vi "Configure Trend Scale.vi"(0 "VISA resource name":refnum<visa-resource-name>, 5 "Scale Digit (0 : Normal)":i32(ring) items=["Normal", "Fine"], 7 "Value Display (0 : Mark)":i32(ring) items=["Mark", "Bar graph"], 9 "digit (0: 0-digit)":i32(ring) items=["0-Digit"=0, "3-Digit"=3, "4-Digit"=4], 11 "error in (no error)":errorcluster) -> (4 "VISA resource name out":refnum<visa-resource-name>, 15 "error out":errorcluster)   [LabVIEW 2020, in "Yokogawa GX Series.lvlib"]
doc: "Sets the scale.\n\nCommand: STrdScale\n\nNote: This VI does nothing when the instrument is GM10."
uses:
  <instrlib>/Yokogawa GX Series/Yokogawa GX Series.lvlib
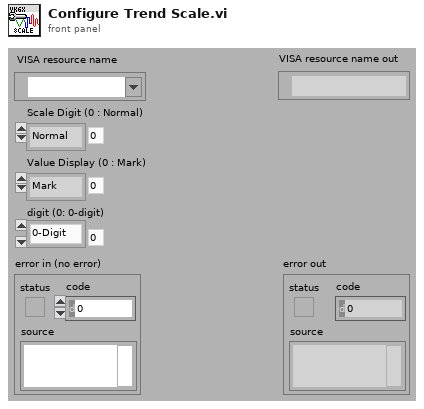
[diagram p1: front panel]
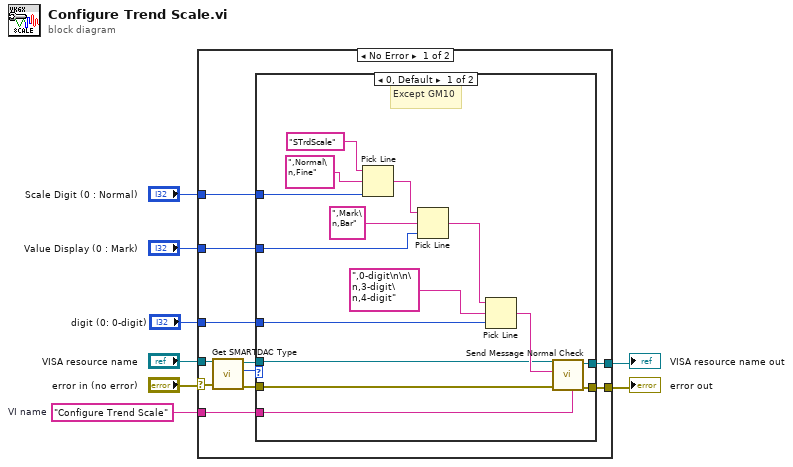
[diagram p0: block diagram]
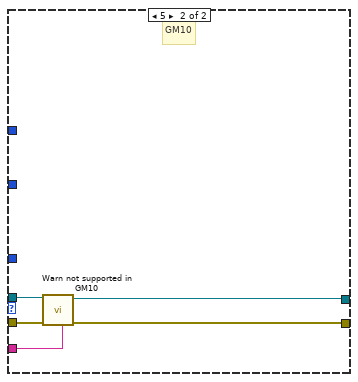
[diagram p2: hidden frame]
diagram:
  w5 = "Configure Trend Scale"  # VI name
  n1 = case shown="No Error" "error in (no error)" {
    selector: "error in (no error)" -> [w12 w40]
    tunnel: "Scale Digit (0 : Normal)" -> [w19 _]
    tunnel: "Value Display (0 : Mark)" -> [w18 _]
    tunnel: "digit (0: 0-digit)" -> [w17 _]
    tunnel: w5 -> [w16 _]
    tunnel: "VISA resource name" -> [w13 w41]
    tunnel: [w15 w41] -> w3
    tunnel: [w14 w40] -> w2
    frame No Error {
      n2 = call <instrlib>:"Get SMARTDAC Type.vi"("error in (no error)"=w12, "VISA resource name"=w13) -> ("error out"=w10:errorcluster, "SMARTDAC+ Type"=w9:u16, "VISA resource name out"=w11:refnum<visa-resource-name>)  [unwired: 7 in]
      n3 = case shown="0, Default" w9 {
        tunnel: w19 -> [w33 _]
        tunnel: w18 -> [w31 _]
        tunnel: w17 -> [w21 _]
        tunnel: w16 -> [w25 w35]
        tunnel: w11 -> [w24 w39]
        tunnel: [w23 w37] -> w15
        tunnel: [w22 w36] -> w14
        tunnel: w10 -> [w20 w38]
        frame 0, Default {
          # "Except GM10"
          n4 = Pick Line(string ("")="STrdScale", multi-line string=",Normal\n,Fine", line index=w33) -> (output string=w30:string)
          n5 = Pick Line(string ("")=w30, multi-line string=",Mark\n,Bar", line index=w31) -> (output string=w28:string)
          n6 = Pick Line(string ("")=w28, multi-line string=",0-digit\n\n\n,3-digit\n,4-digit", line index=w21) -> (output string=w26:string)
          n7 = call <instrlib>:"Send Message Normal Check.vi"("Source (\"\")"=w25, "error in (no error)"=w20, "Send Message (\"\")"=w26, "VISA resource name"=w24) -> ("error out"=w22:errorcluster, "VISA resource name out"=w23:refnum<visa-resource-name>)  [unwired: 2 in, 4 out]
        }
        frame 5 {
          # "GM10"
          n8 = call <instrlib>:"Warn not supported in GM10.vi"("Source (\"\")"=w35, "error in (no error)"=w38, "VISA resource name"=w39) -> ("error out"=w36:errorcluster, "VISA resource name out"=w37:refnum<visa-resource-name>)  [unwired: 7 in]
        }
      }
    }
    frame Error {
    }
  }
  "error out" <- w2
  "VISA resource name out" <- w3
